vi "Reduce Timeout.vi"(8 "error in (no error)":errorcluster, 10 "New Timeout time(ms)":i32, 11 "Response Msg in":refnum<class "Response Msg.lvclass">) -> (0 "error out":errorcluster, 1 "Timeout time reduced?":bool, 3 "Response Msg out":refnum<class "Response Msg.lvclass">)   [LabVIEW 2020, in "Publisher.lvlib" / "Response Msg.lvclass"]
doc: "Reduce the timeout time on the Response Core if possible."
uses:
  Response Msg.lvclass
  Response Msg.lvclass/Response Msg.ctl
  Response Core/Response Core/Response Core.lvclass
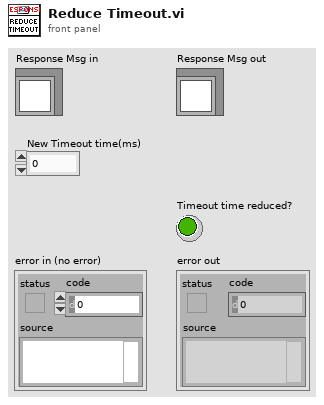
[diagram p1: front panel]
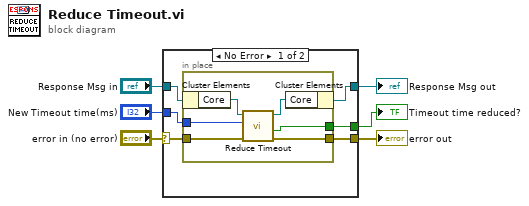
[diagram p0: block diagram]
diagram:
  n1 = case shown="No Error" "error in (no error)" {
    selector: "error in (no error)" -> [w8 w20]
    tunnel: [w7 w20] -> w5
    tunnel: [w11 w19] -> w3
    tunnel: "Response Msg in" -> [w12 w19]
    tunnel: "New Timeout time(ms)" -> [w10 _]
    tunnel: [w9 _] -> w1
    frame No Error {
      n2 = in-place {
        in-place-border: w10 -> [w17]
        in-place-border: [w16] -> w9
        in-place-border: w8 -> [w14]
        in-place-border: [w13] -> w7
        n3 = in-place-cluster #1(w12) -> ("Core"=w18:refnum<class "Response Core.lvclass">)
        n4 = call-dynamic "Reduce Timeout.vi"("error in (no error)"=w14, "New Timeout time(ms)"=w17, "Response Core in"=w18) -> ("error out"=w13:errorcluster, "Timeout time reduced?"=w16:bool, "Response Core out"=w15:refnum<class "Response Core.lvclass">)  [unwired: 6 in]
        n5 = in-place-cluster #1("Core"=w15) -> (w11:refnum<class "Response Msg.lvclass">)
      }
    }
    frame Error {
    }
  }
  "error out" <- w5
  "Response Msg out" <- w3
  "Timeout time reduced?" <- w1
